vi "hse-application_SystemConfiguration_ValidateFile.vi"(8 "error in (no error)":errorcluster, 11 "Config File":path) -> (0 "error out":errorcluster)   [LabVIEW 2022 SP3, in "hse-application.lvclass"]
doc: "Check if <b>Config File</b> exists. If it can't be read, try and copy config.ini.default over to config. ini and show a message. If that also doesn't work, throw an error and show a message.\n\n____\nHAMPEL SOFTWARE ENGINEERING v3.8.0 (2023-12-18 14:41)"
uses:
  hse-application.lvclass
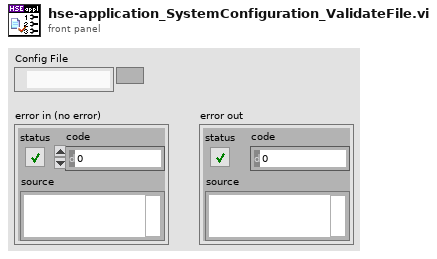
[diagram p1: front panel]
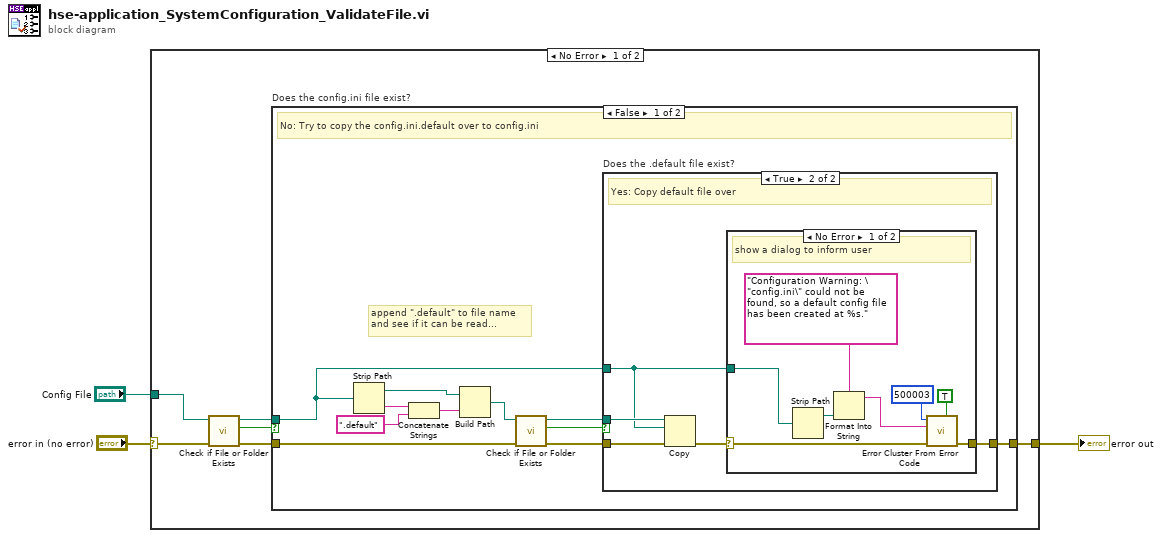
[diagram p0: block diagram]
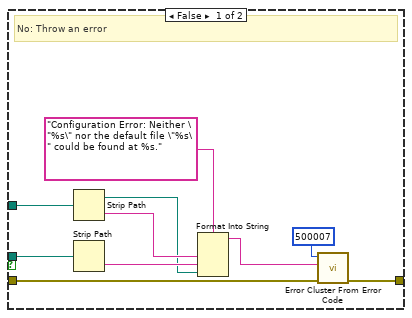
[diagram p2: hidden frame]
diagram:
  n1 = case shown="No Error" "error in (no error)" {
    selector: "error in (no error)" -> [w8 w46]
    tunnel: [w5 w46] -> w2
    tunnel: "Config File" -> [w9 _]
    frame No Error {
      n2 = call <vilib>:"Check if File or Folder Exists.vi"("error in (no error)"=w8, "path"=w9) -> ("error out"=w6:errorcluster, "file or folder exists?"=w7:bool, "dup path"=w4:path)  [unwired: 7 in]
      n3 = case "Does the config.ini file exist?" shown="False" w7 {
        tunnel: w6 -> [w15 w45]
        tunnel: [w10 w45] -> w5
        tunnel: w4 -> [w11 _]
        frame False {
          # "append \".default\" to file name\nand see if it can be read..."
          # "No: Try to copy the config.ini.default over to config.ini"
          n4 = Strip Path(path=w11) -> (stripped path=w19:path, name=w20:string)
          n5 = Concatenate Strings(w20, ".default" ("string")) -> (w18:string)
          n6 = Build Path(base path=w19, name or relative path=w18) -> (appended path=w16:path)
          n7 = call <vilib>:"Check if File or Folder Exists.vi"("error in (no error)"=w15, "path"=w16) -> ("error out"=w14:errorcluster, "file or folder exists?"=w13:bool, "dup path"=w12:path)  [unwired: 7 in]
          n8 = case "Does the .default file exist?" shown="True" w13 {
            tunnel: w14 -> [w23 w35]
            tunnel: w12 -> [w28 w34]
            tunnel: w11 -> [w29 w31]
            tunnel: [w22 w32] -> w10
            frame False {
              # "No: Throw an error"
              n9 = Strip Path(path=w29) -> (stripped path=w25:path, name=w26:string)
              n10 = Strip Path(path=w28) -> (name=w27:string)  [unwired: 1 out]
              n11 = Format Into String(format string="Configuration Error: Neither \"%s\" nor the default file \"%s\" could be found at %s.", w26, w27, w25) -> (resulting string=w21:string)  [unwired: 2 in, 1 out]
              n12 = call <vilib>:"Error Cluster From Error Code.vi"("error in (no error)"=w23, "error message (\"\")"=w21, "error code (0)"=500007) -> ("error out"=w22:errorcluster)  [unwired: 6 in]
            }
            frame True {
              # "Yes: Copy default file over"
              n13 = Copy(8:w35, 10:w31, 11:w34) -> (0:w33:errorcluster)  [unwired: 2 in, 2 out]
              n14 = case shown="No Error" w33 {
                selector: w33 -> [w43 w44]
                tunnel: [w39 w44] -> w32
                tunnel: w31 -> [w41 _]
                frame No Error {
                  # "show a dialog to inform user"
                  n15 = Strip Path(path=w41) -> (stripped path=w40:path)  [unwired: 1 out]
                  n16 = Format Into String(format string="Configuration Warning: \"config.ini\" could not be found, so a default config file has been created at %s.", w40) -> (resulting string=w36:string)  [unwired: 2 in, 1 out]
                  n17 = call <vilib>:"Error Cluster From Error Code.vi"("is warning? (False)"=TRUE, "error in (no error)"=w43, "error message (\"\")"=w36, "error code (0)"=500003) -> ("error out"=w39:errorcluster)  [unwired: 5 in]
                }
                frame Error {
                }
              }
            }
          }
        }
        frame True {
          # "Yes: Do nothing."
        }
      }
    }
    frame Error {
    }
  }
  "error out" <- w2
